vi "CreateTerminalVoltageLogString.vi"(11 "Terminal Voltage (MeV)":dbl) -> (3 "Terminal Voltage Log String":string)   [LabVIEW 2012]
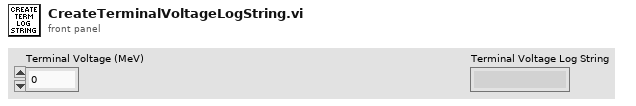
[diagram p1: front panel]
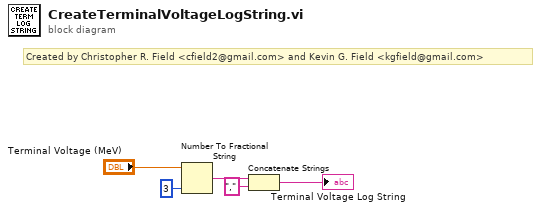
[diagram p0: block diagram]
diagram:
  # "Created by Christopher R. Field <cfield2@gmail.com> and Kevin G. Field <kgfield@gmail.com>"
  n1 = Number To Fractional String(number="Terminal Voltage (MeV)", precision (6)=i16 3) -> (F-format string=w3:string)  [unwired: 2 in]
  n2 = Concatenate Strings(w3, "," ("string")) -> (→"Terminal Voltage Log String":string)
